vi "TP 4.1 (no programable).vi"() -> ()   [LabVIEW 2013]
uses:
  <vilib>/gmath/statdist.llb/Normal Inverse CDF.vi
  <vilib>/gmath/NI_Gmath.lvlib
panel:
  out "Waveform Chart":cluster{"x":dbl, dbl}(graph)
  in  "stop":bool
  in  "Nivel de ruido":dbl=2.0
  in  "Medicion":dbl=10.0
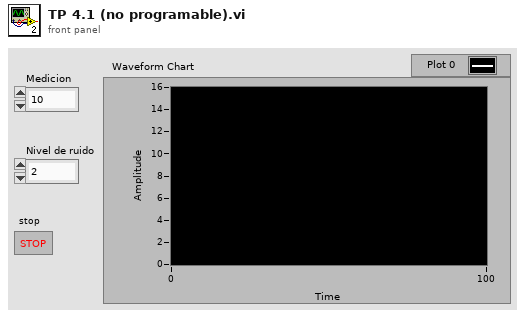
[diagram p1: front panel]
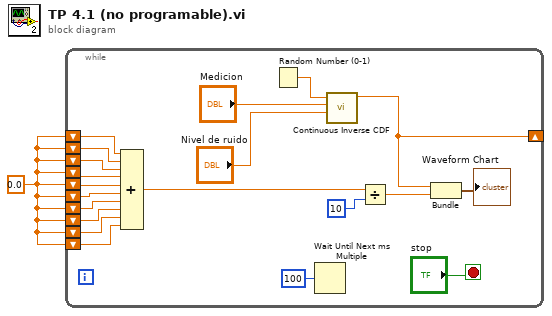
[diagram p0: block diagram]
diagram:
  w1 = 0.0 ("element")
  n1 = while {
    shift-right: [w2] -> _
    shift-left: w1 -> [w13]
    shift-left: w1 -> [w12]
    shift-left: w1 -> [w11]
    shift-left: w1 -> [w10]
    shift-left: w1 -> [w9]
    shift-left: w1 -> [w8]
    shift-left: w1 -> [w4]
    shift-left: w1 -> [w7]
    shift-left: w1 -> [w6]
    shift-left: w1 -> [w5]
    stop <- "stop" stop-if-true
    n2 = Compound Arithmetic op=ADD(w13, w12, w11, w10, w9, w8, w4, w7, w6, w5) -> (w3:dbl)
    n3 = Random Number (0-1)() -> (number: 0 to 1=w19:dbl)
    n4 = Wait Until Next ms Multiple(millisecond multiple=u32 100) -> ()  [unwired: 1 out]
    n5 = call-poly <vilib>:"Continuous Inverse CDF.vi"("std"="Nivel de ruido", "mean"="Medicion", "cdf(x)"=w19) -> ("x"=w2:dbl)  [unwired: 7 in, 1 out]
    n6 = Divide(x=w3, y=10) -> (x/y=w17:dbl)
    n7 = Bundle("x"=w2, w17) -> (→"Waveform Chart":cluster{"x":dbl, dbl})  [unwired: 1 in]
  }
